vi "Teleop.vi"(10 "Match Info":T1={"Autonomous Elapsed Seconds"=0.0, "TeleOp Elapsed Seconds"=0.0, "Disabled Elapsed Seconds"=0.0, "Visited Autonomous"=FALSE, "Visited TeleOp"=FALSE, "Visited Disabled"=FALSE, "Autonomous Settings"={"Autonomous Style"=enum."Independent", "VI Refnum"=refnum}}, 11 "Call Context":T2) -> ()   [LabVIEW 2019]
doc: "This VI is called for each TeleOp packet received from the DS where the robot is not disabled. It is often used to read from the joysticks and update I/O or to update setpoints for timed control loops. It should complete and return within 20 milliseconds or it may miss DS packets."
uses:
  <vilib>/Rock Robotics/Network Tables/NT Write Numeric Array.vi
  Robot Global Data.vi
  Control 1.ctl
  <vilib>/Rock Robotics/WPI/RobotDrive/WPI_RobotDriveMecanumDrive_Cartesian.vi
  <vilib>/Rock Robotics/Network Tables/NT Read Boolean.vi
  <vilib>/Rock Robotics/Network Tables/NT Read Number.vi
  <vilib>/Rock Robotics/Network Tables/NT Write Boolean Array.vi
  <vilib>/Rock Robotics/WPI/DriverStation/WPI_DriverStationMatch Info.ctl
  <vilib>/Rock Robotics/WPI/DriverStation/WPI_DriverStationDerivedRobotMode.ctl
panel:
  out "Didit":bool
  out "Sample Slider 0":dbl(slide) scale=0.0..5.0
  out "Sample Boolean 1":bool
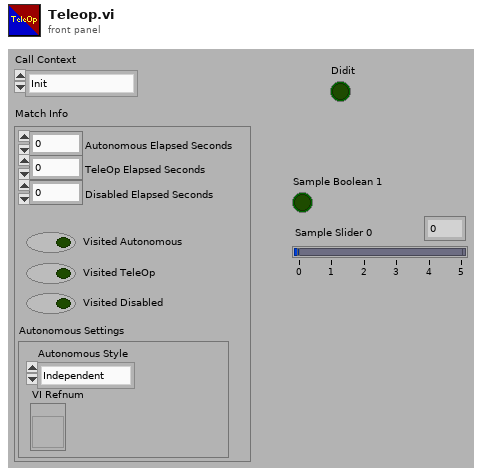
[diagram p1: front panel]
types:
  T1 = typedef "WPI_DriverStationMatch Info.ctl" = cluster{"Autonomous Elapsed Seconds":dbl, "TeleOp Elapsed Seconds":dbl, "Disabled Elapsed Seconds":dbl, "Visited Autonomous":bool, "Visited TeleOp":bool, "Visited Disabled":bool, "Autonomous Settings":cluster{"Autonomous Style":enum16{"Iterative", "Independent"}, "VI Refnum":refnum<vi>}}
  T2 = typedef "WPI_DriverStationDerivedRobotMode.ctl" = enum16{"Init", "Execute", "Stop"}
  T3 = typedef "WPI_RobotDriveDevRef.ctl" = cluster{"DevStatus":errorcluster, "Motors[]":T4[], "Square Inputs":bool, "Max Output":dbl}
  T4 = typedef "WPI_MotorControlDeviceRef.ctl" = cluster{"DeviceStatus":errorcluster, "Type":T5, "PWM":cluster{"PWM Channel":T6, "DeadBand":T7}, "CAN":cluster{"Device Number":u8, "SetOutput VI Ref":variant, "GetOutput VI Ref":variant, "Enable VI Ref":variant, "Disable VI Ref":variant, "Data":variant}, "Invert":bool, "DIO PWM":cluster{"PWM \"Enable\" Channel":T6, "DIOChannel":T8, "PWM Rate":dbl}}
  T5 = typedef "WPI_MotorControlType.ctl" = enum16{"PWM", "CAN", "DIO PWM"}
  T6 = typedef "FPGA_DIOPWMChannel.ctl" = enum8{"PWM 0", "PWM 1", "PWM 2", "PWM 3", "PWM 4", "PWM 5", "PWM 6", "PWM 7", "PWM 8", "PWM 9", "PWM MXP 0", "PWM MXP 1", "PWM MXP 2", "PWM MXP 3", "PWM MXP 4", "PWM MXP 5", "PWM MXP 6", "PWM MXP 7", "PWM MXP 8", "PWM MXP 9", "Invalid"}
  T7 = typedef "WPI_PWMDeadband.ctl" = cluster{"Name":string, "maxPositivePwm":i32, "minPositivePwm":i32, "centerPwm":i32, "maxNegativePwm":i32, "minNegativePwm":i32, "angularRange":u16}
  T8 = typedef "FPGA_DIOChannel.ctl" = enum8{"DIO 0", "DIO 1", "DIO 2", "DIO 3", "DIO 4", "DIO 5", "DIO 6", "DIO 7", "DIO 8", "DIO 9", "DIO MXP 0", "DIO MXP 1", "DIO MXP 2", "DIO MXP 3", "DIO MXP 4", "DIO MXP 5", "DIO MXP 6", "DIO MXP 7", "DIO MXP 8", "DIO MXP 9", "DIO MXP 10", "DIO MXP 11", "DIO MXP 12", "DIO MXP 13", "DIO MXP 14", "DIO MXP 15", "SPI Port CS1", "SPI Port CS2", "SPI Port CS3", "SPI Port MISO", "SPI Port MOSI", "Invalid"}
  T9 = typedef "WPI_JoystickDevRef.ctl" = cluster{"Device":T10}
  T10 = typedef "WPI_JoystickDeviceEnum.ctl" = enum16{"USB 0", "USB 1", "USB 2", "USB 3", "USB 4", "USB 5"}
  T11 = typedef "Color Sensor V3 DevRef.ctl" = cluster{"I2CDevRef":T12}
  T12 = typedef "WPI_I2CDevRef.ctl" = cluster{"DevStatus":errorcluster, "Device Address":u8, "Handle":i32, "I2C Bus":T13}
  T13 = typedef "i2c_bus.ctl" = enum16{"I2C On-Board", "I2C MXP", "Invalid"}
  T14 = typedef "Control 1.ctl" = bool
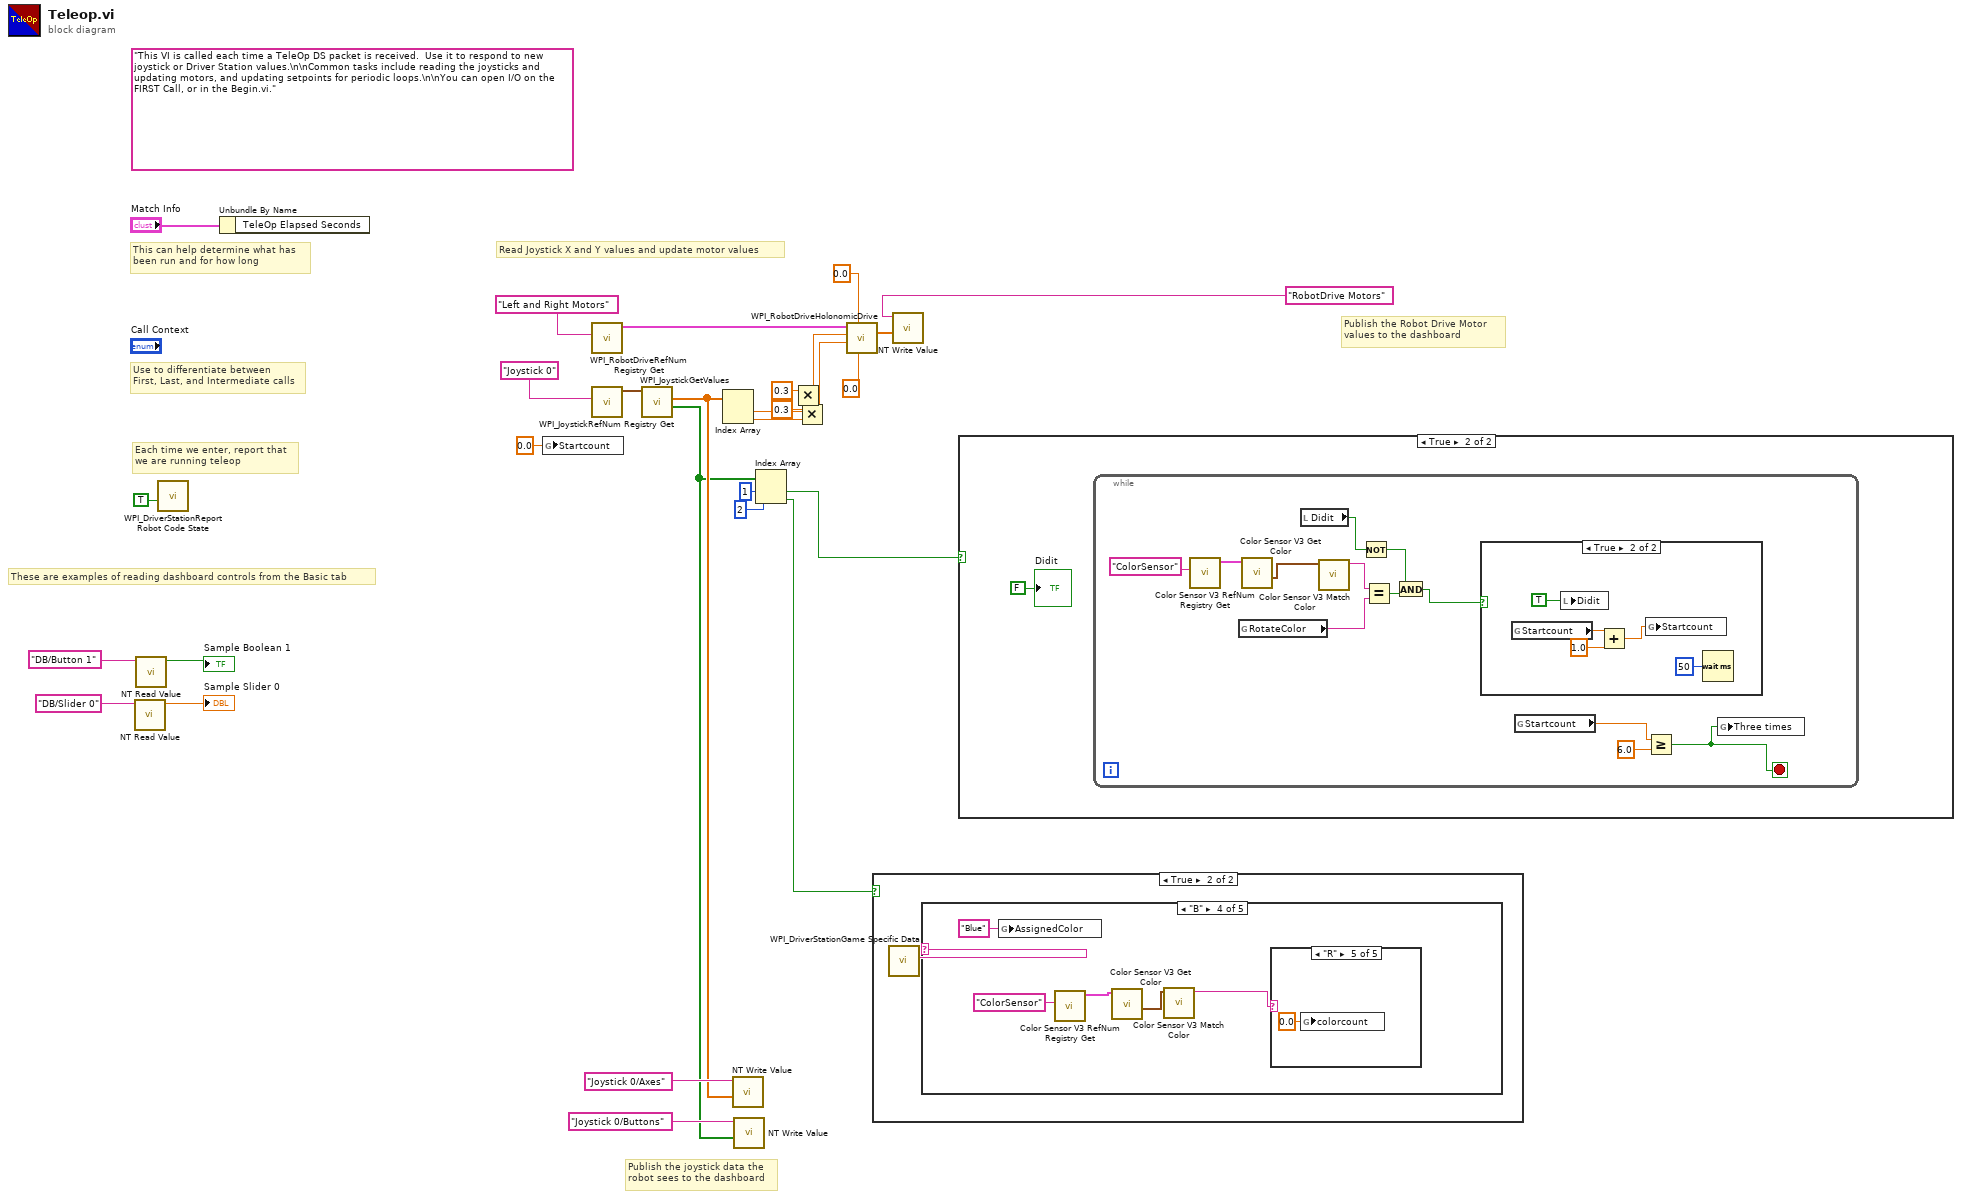
[diagram p0: block diagram]
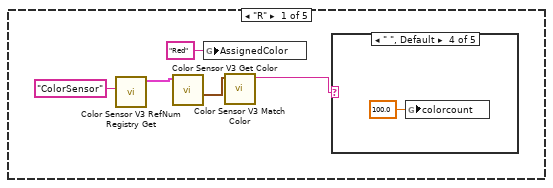
[diagram p3: hidden frame]
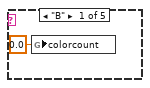
[diagram p4: hidden frame]
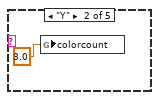
[diagram p5: hidden frame]
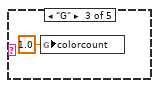
[diagram p6: hidden frame]
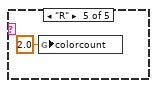
[diagram p7: hidden frame]
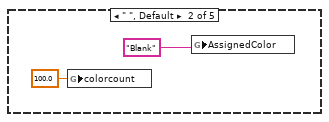
[diagram p8: hidden frame]
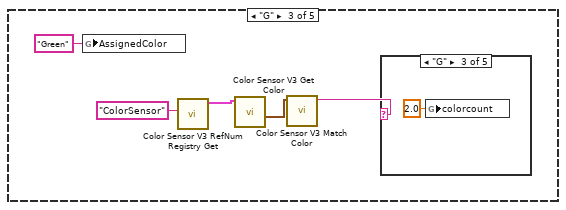
[diagram p9: hidden frame]
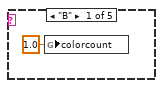
[diagram p10: hidden frame]
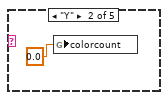
[diagram p11: hidden frame]
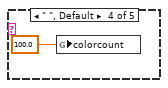
[diagram p12: hidden frame]
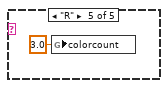
[diagram p13: hidden frame]
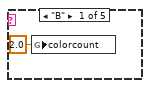
[diagram p14: hidden frame]
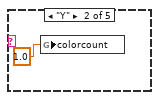
[diagram p15: hidden frame]
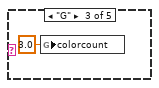
[diagram p16: hidden frame]
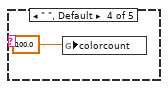
[diagram p17: hidden frame]
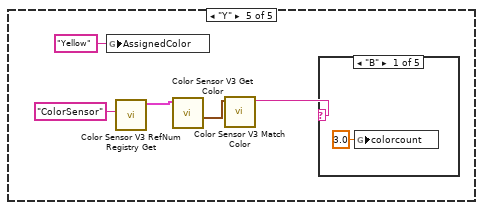
[diagram p18: hidden frame]
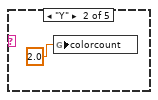
[diagram p19: hidden frame]
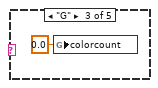
[diagram p20: hidden frame]
diagram:
  (unwired) "This VI is called each time a TeleOp DS packet is received.  Use it to respond to new joystick or Driver Station values.\n\nCommon tasks include reading the joysticks and updating motors, and updating setpoints for periodic loops.\n\nYou can open I/O on the FIRST Call, or in the Begin.vi."
  # "These are examples of reading dashboard controls from the Basic tab"
  # "Publish the Robot Drive Motor\nvalues to the dashboard"
  # "Publish the joystick data the\nrobot sees to the dashboard"
  # "Each time we enter, report that\nwe are running teleop"
  # "Use to differentiate between\nFirst, Last, and Intermediate calls"
  # "This can help determine what has\nbeen run and for how long"
  # "Read Joystick X and Y values and update motor values"
  n1 = call-poly <vilib>:"NT Read Value.vi"("Name"="DB/Slider 0" ("refnum name")) -> ("Numeric"=→"Sample Slider 0":dbl)  [unwired: 9 in, 1 out]
  n2 = call-poly <vilib>:"NT Read Value.vi"("Name"="DB/Button 1" ("refnum name")) -> ("Boolean"=→"Sample Boolean 1":bool)  [unwired: 9 in, 1 out]
  n3 = call <vilib>:"WPI_DriverStationReport Robot Code State.vi"("TeleOp"=TRUE ("Autonomous")) -> ()  [unwired: 10 in, 1 out]
  n4 = Unbundle By Name("Match Info") -> ()  [unwired: 1 out]
  n5 = global write "Robot Global Data.vi" "Startcount"(0.0 ("Startcount")) -> ()
  n6 = call <vilib>:"WPI_RobotDriveRefNum Registry Get.vi"("refnum name"="Left and Right Motors") -> ("RobotDriveDevRef"=w27:T3)  [unwired: 1 in, 9 out]
  n7 = call <vilib>:"WPI_JoystickRefNum Registry Get.vi"("refnum name"="Joystick 0") -> ("JoystickDevRef"=w24:T9)  [unwired: 1 in, 9 out]
  n8 = call <vilib>:"WPI_JoystickGetValues.vi"("JoystickDevRef"=w24) -> ("Buttons"=w6:bool[], "Axes"=w19:dbl[])  [unwired: 6 in, 3 out]
  n9 = Index Array(array=w19) -> (element #1=w26:dbl, element #2=w22:dbl)  [unwired: 2 in]
  n10 = call-poly <vilib>:"NT Write Value.vi"("Numeric Array"=w19, "Name"="Joystick 0/Axes") -> ()  [unwired: 9 in, 1 out]
  n11 = call-poly <vilib>:"NT Write Value.vi"("Boolean Array"=w6, "Name"="Joystick 0/Buttons") -> ()  [unwired: 9 in, 1 out]
  n12 = Index Array(array=w6, index #1=1 ("index"), index #2=2 ("index")) -> (element #1=w4:bool, element #2=w1:bool)
  n13 = Multiply(x=0.3, y=w26) -> (x*y=w10:dbl)
  n14 = Multiply(x=0.3, y=w22) -> (x*y=w8:dbl)
  n15 = call-poly <vilib>:"WPI_RobotDriveHolonomicDrive.vi"("Rotation"=0.0, "Gyro Angle"=0.0, "Y"=w8, "X"=w10, "RobotDriveDevRef"=w27) -> ("Motor Values"=w14:dbl[])  [unwired: 4 in, 2 out]
  n16 = case shown="True" w1 {
    frame False {
    }
    frame True {
      n17 = call <vilib>:"WPI_DriverStationGame Specific Data.vi"() -> ("Game Specific Data"=w30:string)  [unwired: 11 in]
      n18 = case shown="\"B\"" w30 {
        frame "R" {
          n19 = call <vilib>:"Color Sensor V3 RefNum Registry Get.vi"("refnum name"="ColorSensor") -> ("ColorSensorDevRef"=w33:T11)  [unwired: 9 in, 1 out]
          n20 = call <vilib>:"Color Sensor V3 Get Color.vi"("ColorSensorDevRef"=w33) -> ("Normalized Color"=w32:cluster{"R":dbl, "G":dbl, "B":dbl})  [unwired: 7 in, 3 out]
          n21 = global write "Robot Global Data.vi" "AssignedColor"("Red" ("AssignedColor")) -> ()
          n22 = call <vilib>:"Color Sensor V3 Match Color.vi"("Measured Color"=w32) -> ("Matched Color Name"=w31:string)  [unwired: 8 in, 2 out]
          n23 = case shown="\" \", Default" w31 {
            frame "B" {
              n24 = global write "Robot Global Data.vi" "colorcount"(0.0 ("colorcount")) -> ()
            }
            frame "Y" {
              n25 = global write "Robot Global Data.vi" "colorcount"(3.0 ("colorcount")) -> ()
            }
            frame "G" {
              n26 = global write "Robot Global Data.vi" "colorcount"(1.0 ("colorcount")) -> ()
            }
            frame " ", Default {
              n27 = global write "Robot Global Data.vi" "colorcount"(100.0 ("colorcount")) -> ()
            }
            frame "R" {
              n28 = global write "Robot Global Data.vi" "colorcount"(2.0 ("colorcount")) -> ()
            }
          }
        }
        frame " ", Default {
          n29 = global write "Robot Global Data.vi" "colorcount"(100.0 ("colorcount")) -> ()
          n30 = global write "Robot Global Data.vi" "AssignedColor"("Blank" ("AssignedColor")) -> ()
        }
        frame "G" {
          n31 = global write "Robot Global Data.vi" "AssignedColor"("Green" ("AssignedColor")) -> ()
          n32 = call <vilib>:"Color Sensor V3 RefNum Registry Get.vi"("refnum name"="ColorSensor") -> ("ColorSensorDevRef"=w45:T11)  [unwired: 9 in, 1 out]
          n33 = call <vilib>:"Color Sensor V3 Get Color.vi"("ColorSensorDevRef"=w45) -> ("Normalized Color"=w44:cluster{"R":dbl, "G":dbl, "B":dbl})  [unwired: 7 in, 3 out]
          n34 = call <vilib>:"Color Sensor V3 Match Color.vi"("Measured Color"=w44) -> ("Matched Color Name"=w43:string)  [unwired: 8 in, 2 out]
          n35 = case shown="\"G\"" w43 {
            frame "B" {
              n36 = global write "Robot Global Data.vi" "colorcount"(1.0 ("colorcount")) -> ()
            }
            frame "Y" {
              n37 = global write "Robot Global Data.vi" "colorcount"(0.0 ("colorcount")) -> ()
            }
            frame "G" {
              n38 = global write "Robot Global Data.vi" "colorcount"(2.0 ("colorcount")) -> ()
            }
            frame " ", Default {
              n39 = global write "Robot Global Data.vi" "colorcount"(100.0 ("colorcount")) -> ()
            }
            frame "R" {
              n40 = global write "Robot Global Data.vi" "colorcount"(3.0 ("colorcount")) -> ()
            }
          }
        }
        frame "B" {
          n41 = global write "Robot Global Data.vi" "AssignedColor"("Blue" ("AssignedColor")) -> ()
          n42 = call <vilib>:"Color Sensor V3 RefNum Registry Get.vi"("refnum name"="ColorSensor") -> ("ColorSensorDevRef"=w55:T11)  [unwired: 9 in, 1 out]
          n43 = call <vilib>:"Color Sensor V3 Get Color.vi"("ColorSensorDevRef"=w55) -> ("Normalized Color"=w54:cluster{"R":dbl, "G":dbl, "B":dbl})  [unwired: 7 in, 3 out]
          n44 = call <vilib>:"Color Sensor V3 Match Color.vi"("Measured Color"=w54) -> ("Matched Color Name"=w53:string)  [unwired: 8 in, 2 out]
          n45 = case shown="\"R\"" w53 {
            frame "B" {
              n46 = global write "Robot Global Data.vi" "colorcount"(2.0 ("colorcount")) -> ()
            }
            frame "Y" {
              n47 = global write "Robot Global Data.vi" "colorcount"(1.0 ("colorcount")) -> ()
            }
            frame "G" {
              n48 = global write "Robot Global Data.vi" "colorcount"(3.0 ("colorcount")) -> ()
            }
            frame " ", Default {
              n49 = global write "Robot Global Data.vi" "colorcount"(100.0 ("colorcount")) -> ()
            }
            frame "R" {
              n50 = global write "Robot Global Data.vi" "colorcount"(0.0 ("colorcount")) -> ()
            }
          }
        }
        frame "Y" {
          n51 = global write "Robot Global Data.vi" "AssignedColor"("Yellow" ("AssignedColor")) -> ()
          n52 = call <vilib>:"Color Sensor V3 RefNum Registry Get.vi"("refnum name"="ColorSensor") -> ("ColorSensorDevRef"=w65:T11)  [unwired: 9 in, 1 out]
          n53 = call <vilib>:"Color Sensor V3 Get Color.vi"("ColorSensorDevRef"=w65) -> ("Normalized Color"=w64:cluster{"R":dbl, "G":dbl, "B":dbl})  [unwired: 7 in, 3 out]
          n54 = call <vilib>:"Color Sensor V3 Match Color.vi"("Measured Color"=w64) -> ("Matched Color Name"=w63:string)  [unwired: 8 in, 2 out]
          n55 = case shown="\"B\"" w63 {
            frame "B" {
              n56 = global write "Robot Global Data.vi" "colorcount"(3.0 ("colorcount")) -> ()
            }
            frame "Y" {
              n57 = global write "Robot Global Data.vi" "colorcount"(2.0 ("colorcount")) -> ()
            }
            frame "G" {
              n58 = global write "Robot Global Data.vi" "colorcount"(0.0 ("colorcount")) -> ()
            }
            frame " ", Default {
              n59 = global write "Robot Global Data.vi" "colorcount"(100.0 ("colorcount")) -> ()
            }
            frame "R" {
              n60 = global write "Robot Global Data.vi" "colorcount"(1.0 ("colorcount")) -> ()
            }
          }
        }
      }
    }
  }
  n61 = call-poly <vilib>:"NT Write Value.vi"("Numeric Array"=w14, "Name"="RobotDrive Motors") -> ()  [unwired: 9 in, 1 out]
  n62 = case shown="True" w4 {
    frame False {
    }
    frame True {
      n63 = while {
        stop <- w77 stop-if-true
        n64 = call <vilib>:"Color Sensor V3 RefNum Registry Get.vi"("refnum name"="ColorSensor") -> ("ColorSensorDevRef"=w84:T11)  [unwired: 9 in, 1 out]
        n65 = global read "Robot Global Data.vi" "RotateColor"() -> (w74:string)
        n66 = call <vilib>:"Color Sensor V3 Get Color.vi"("ColorSensorDevRef"=w84) -> ("Normalized Color"=w76:cluster{"R":dbl, "G":dbl, "B":dbl})  [unwired: 7 in, 3 out]
        n67 = local read "Didit"() -> (w82:bool)
        n68 = call <vilib>:"Color Sensor V3 Match Color.vi"("Measured Color"=w76) -> ("Matched Color Name"=w75:string)  [unwired: 8 in, 2 out]
        n69 = Not(x=w82) -> (.not. x?=w81:bool)
        n70 = Equal?(x=w75, y=w74) -> (x = y?=w83:bool)
        n71 = And(x=w81, y=w83) -> (x .and. y?=w80:bool)
        n72 = case shown="True" w80 {
          frame False {
            n73 = local write "Didit"(T14 FALSE ("Didit 2")) -> ()
          }
          frame True {
            n74 = global read "Robot Global Data.vi" "Startcount"() -> (w90:dbl)
            n75 = local write "Didit"(T14 TRUE ("Didit 2")) -> ()
            n76 = Add(x=w90, y=1.0) -> (x+y=w88:dbl)
            n77 = global write "Robot Global Data.vi" "Startcount"(w88) -> ()
            n78 = Wait (ms)(milliseconds to wait=u32 50) -> ()  [unwired: 1 out]
          }
        }
        n79 = global read "Robot Global Data.vi" "Startcount"() -> (w79:dbl)
        n80 = Greater Or Equal?(x=w79, y=6.0) -> (x >= y?=w77:bool)
        n81 = global write "Robot Global Data.vi" "Three times"(w77) -> ()
      }
      "Didit" <- FALSE ("Didit")
    }
  }
